vi "Read ToolStrip.vi"(8 "error in (no error)":errorcluster, 11 "ToolStrip in":refnum<class "MGI_ToolStrip.lvclass">) -> (0 "error out":errorcluster, 2 "ToolStrip":refnum<k24>, 3 "ToolStrip out":refnum<class "MGI_ToolStrip.lvclass">)   [LabVIEW 2019, in "MGI_ToolStrip.lvclass"]
uses:
  MGI_ToolStrip.lvclass
  System.Windows.Forms
  MGI_ToolStrip.lvclass/MGI_ToolStrip.ctl
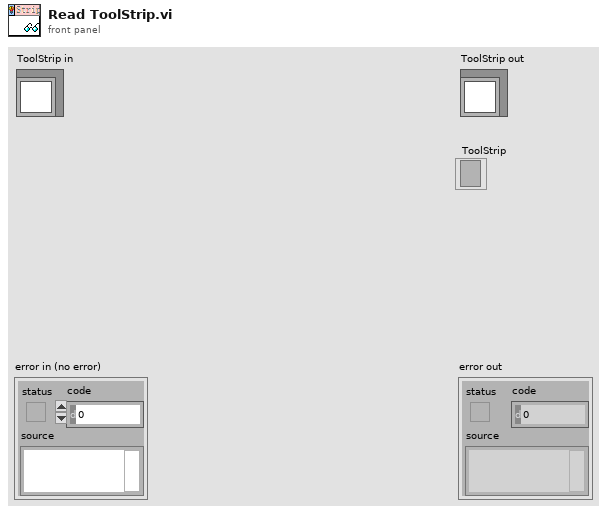
[diagram p1: front panel]
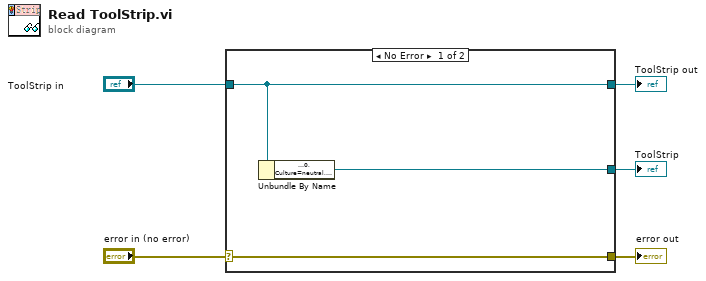
[diagram p0: block diagram]
diagram:
  n1 = case shown="No Error" "error in (no error)" {
    selector: "error in (no error)" -> [w8 w9]
    tunnel: [w8 w9] -> w4
    tunnel: [w7 w10] -> w2
    tunnel: "ToolStrip in" -> [w7 w10]
    tunnel: [w6 _] -> w1
    frame No Error {
      n2 = Unbundle By Name(w7) -> ("ToolStrip"=w6:refnum<k24>)
    }
    frame Error {
    }
  }
  "error out" <- w4
  "ToolStrip out" <- w2
  "ToolStrip" <- w1
